vi "Draw Axes.vi"(8 "Error In (no Error) In":errorcluster, 9 "Show Axes In":bool, 10 "WFGraph Refnum In":refnum<vi>, 11 "Display State In":T1={"Show Axes"=FALSE, "Show Y=0"=FALSE, "Controls"={"Type"=enum."Sine", "Periods"=0.0, "Points"=0, "Offset"=0.0, "Amplitdue"=0.0, "Phase"=0.0, "func"=""}, "Show Current Location"=FALSE, "Current Location"=0, "dt"=0.0, "t0"=timestamp(0 s since 1904-01-01), "Format and Units"="%_3p"} caption="State") -> (0 "Error Out":errorcluster, 3 "Display State Out":T1={"Show Axes"=FALSE, "Show Y=0"=FALSE, "Controls"={"Type"=enum."Sine", "Periods"=0.0, "Points"=0, "Offset"=0.0, "Amplitdue"=0.0, "Phase"=0.0, "func"=""}, "Show Current Location"=FALSE, "Current Location"=0, "dt"=0.0, "t0"=timestamp(0 s since 1904-01-01), "Format and Units"="%_3p"} caption="State")   [LabVIEW 2018, in "Waveform Control.xctl"]
doc: "Turns on/off the axes display on the preview plot"
uses:
  Waveform Control.xctl
  Controls/Waveform State.ctl
  FP Controls.ctl
  Function Types.ctl
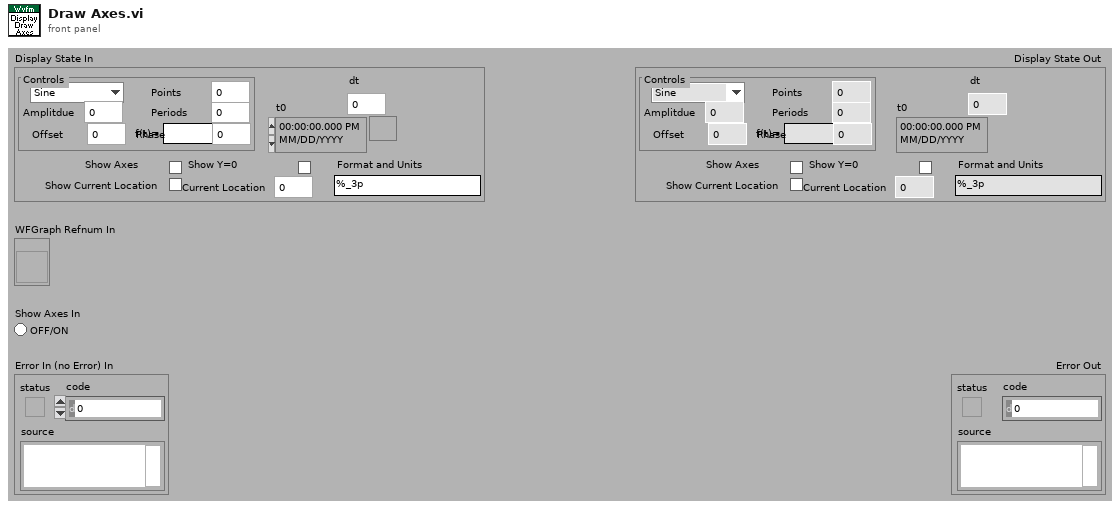
[diagram p1: front panel]
types:
  T1 = typedef "Waveform Control.xctl/Waveform State.ctl" = cluster{"Show Axes":bool, "Show Y=0":bool, "Controls":T2, "Show Current Location":bool, "Current Location":i32, "dt":dbl, "t0":timestamp, "Format and Units":string}
  T2 = typedef "Waveform Control.xctl/FP Controls.ctl" = cluster{"Type":T3, "Periods":dbl, "Points":i32, "Offset":dbl, "Amplitdue":dbl, "Phase":dbl, "func":string}
  T3 = typedef "Waveform Control.xctl/Function Types.ctl" = enum16{"Level", "Sine", "Triangle", "Ramp", "Saw Tooth", "Square", "Function"}
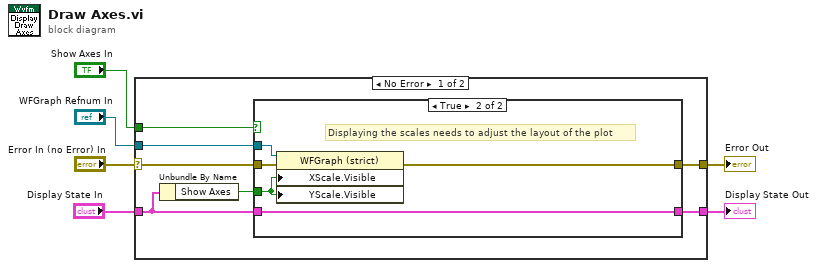
[diagram p0: block diagram]
diagram:
  n1 = case shown="No Error" "Error In (no Error) In" {
    selector: "Error In (no Error) In" -> [w13 w22]
    tunnel: [w12 w22] -> w5
    tunnel: "Show Axes In" -> [w11 _]
    tunnel: "WFGraph Refnum In" -> [w9 _]
    tunnel: [w8 w21] -> w2
    tunnel: "Display State In" -> [w7 w21]
    frame No Error {
      n2 = Unbundle By Name(w7) -> ("Show Axes"=w10:bool)
      n3 = case shown="True" w11 {
        tunnel: w10 -> [_ w20]
        tunnel: [w14 w19] -> w12
        tunnel: w13 -> [w14 w18]
        tunnel: w9 -> [_ w17]
        tunnel: [w15 w16] -> w8
        tunnel: w7 -> [w15 w16]
        frame False {
        }
        frame True {
          # "Displaying the scales needs to adjust the layout of the plot"
          n4 = property on="Property Node" class="WFGraph (strict)"(reference=w17, error in=w18, "XScale.Visible"=w20, "YScale.Visible"=w20) -> (error out=w19:errorcluster)  [unwired: 1 out]
        }
      }
    }
    frame Error {
    }
  }
  "Error Out" <- w5
  "Display State Out" <- w2
